vi "Load Tests.vi"(8 "error in (no error)":errorcluster, 10 "Tests":string[](array[string]), 11 "Execution UI In":refnum<class "Execution UI V2.lvclass">) -> (0 "error out":errorcluster, 3 "Execution UI Out":refnum<class "Execution UI V2.lvclass">)   [LabVIEW 2020]
uses:
  Execution UI V2.lvclass
  Execution UI V2.lvclass/Execution UI V2.ctl
  Framework/Test Suite/LUnit Test Suite.lvclass
  Framework/Test Suite/LUnit Test Suite.lvclass/LUnit Test Suite.ctl
  Framework/Test Case/LUnit Test Case.lvclass/LUnit Test Case.ctl
  Framework/Test Case/Public/Accessors/Read Enabled Test Methods.vi
  C:/Git/astemes-lunit/source/Application Framework/Process Classes/Process/Process.lvclass
  C:/Git/astemes-lunit/source/Rewrite Project/Execution UI/Execution UI V2.lvclass
  Framework/Helper Classes/Test Finder/Test Finder.lvclass
  C:/Git/astemes-lunit/source/Framework/Helper Classes/Test Finder/Test Finder.lvclass
  C:/Git/astemes-lunit/source/Framework/Helper Classes/Open Test Case Interface/Open Test Case.lvclass
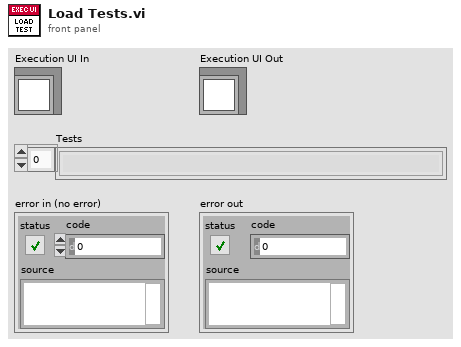
[diagram p1: front panel]
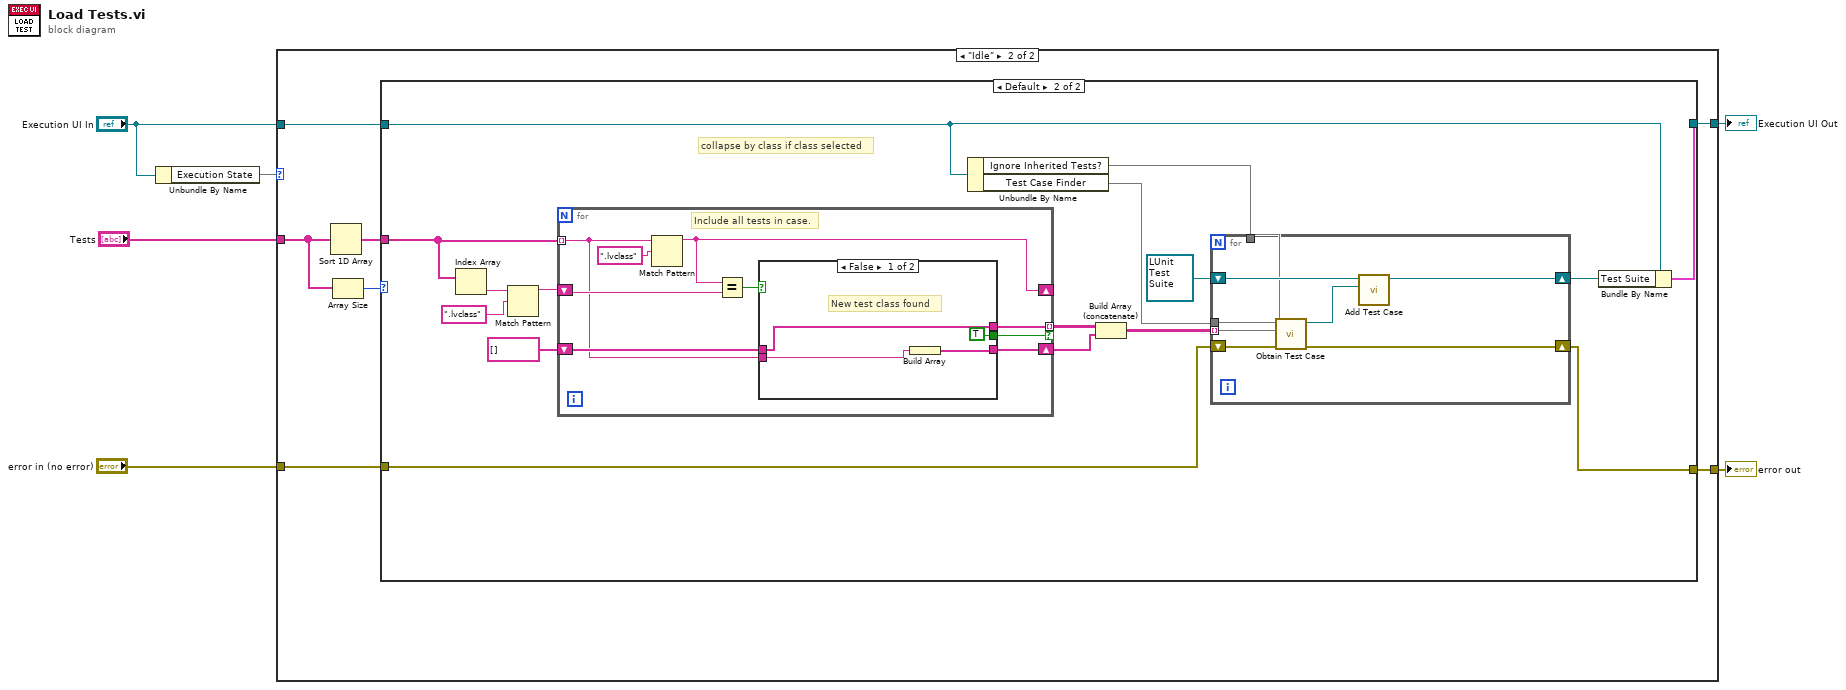
[diagram p0: block diagram]
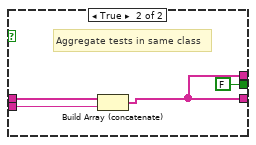
[diagram p4: hidden frame]
diagram:
  n1 = Unbundle By Name("Execution UI In") -> ("Execution State"=w1)
  n2 = case shown="\"Idle\"" w1 {
    tunnel: [w8 w15] -> w6
    tunnel: [w7 w14] -> w5
    tunnel: "error in (no error)" -> [w7 w13]
    tunnel: "Tests" -> [_ w12]
    tunnel: "Execution UI In" -> [w8 w9]
    frame "Running" {
    }
    frame "Idle" {
      n3 = Sort 1D Array(array=w12) -> (sorted array=w10:string[])
      n4 = Array Size(array=w12) -> (size(s)=w11:i32)
      n5 = case shown="Default" w11 {
        tunnel: [w17 w33] -> w15
        tunnel: w9 -> [w17 w20]
        tunnel: [w16 w23] -> w14
        tunnel: w13 -> [w16 w22]
        tunnel: w10 -> [_ w21]
        frame 0 {
        }
        frame Default {
          # "collapse by class if class selected"
          n6 = Index Array(array=w21) -> (element=w27:string)  [unwired: 1 in]
          n7 = Match Pattern(string=w27, regular expression=".lvclass") -> (before substring=w26:string)  [unwired: 1 in, 3 out]
          n8 = for {
            tunnel: w21 -> [w45] mode=indexing
            shift-right: [w48] -> _
            shift-left: w26 -> [w49]
            shift-right: [w44] -> w29
            shift-left: string[] [] ("String") -> [w46]
            tunnel: [w42] -> w31 mode=indexing if=w43
            # "Include all tests in case."
            n9 = Match Pattern(string=w45, regular expression=".lvclass") -> (before substring=w48:string)  [unwired: 1 in, 3 out]
            n10 = Equal?(x=w48, y=w49) -> (x = y?=w47:bool)
            n11 = case shown="False" w47 {
              tunnel: w45 -> [w53 w58]
              tunnel: w46 -> [w51 w57]
              tunnel: [w54 w55] -> w44
              tunnel: [TRUE FALSE] -> w43
              tunnel: [w51 w55] -> w42
              frame False {
                # "New test class found"
                n12 = Build Array(w53) -> (w54:string[])
              }
              frame True {
                # "Aggregate tests in same class"
                n13 = Build Array (concatenate)(w57, w58) -> (w55:string[])
              }
            }
          }
          n14 = Unbundle By Name(w20) -> ("Ignore Inherited Tests?"=w18, "Test Case Finder"=w19)
          n15 = Build Array (concatenate)(w31, w29) -> (w30:string[][])
          n16 = for {
            tunnel: w30 -> [w36] mode=indexing
            shift-right: [w37] -> w24
            shift-left: refnum<class "LUnit Test Suite.lvclass"> refnum ("Test Suite In") -> [w41]
            shift-right: [w35] -> w23
            shift-left: w22 -> [w39]
            tunnel: w19 -> [w38]
            tunnel: w18 -> [w34]
            n17 = call "Obtain Test Case.vi"("error in (no error)"=w39, "Ignore Inherited Tests?"=w34, "Test class and methods"=w36, "Test Finder"=w38) -> ("error out"=w35:errorcluster, "Test Case"=w40:refnum<class "LUnit Test Case.lvclass">)  [unwired: 6 in]
            n18 = call "Add Test Case.vi"("Test Case to add"=w40, "Test Suite In"=w41) -> ("Test Suite Out"=w37:refnum<class "LUnit Test Suite.lvclass">)  [unwired: 9 in]
          }
          n19 = Bundle By Name(cluster=w20, "Test Suite"=w24) -> (w33:cluster{})
        }
      }
    }
  }
  "error out" <- w5
  "Execution UI Out" <- w6
